vi "set_sweep_period.vi"(8 "error in (no error)":errorcluster, 10 "sweep period":dbl[unit], 11 "DL090130ExperimentController.lvclass in":refnum<class "ExperimentControllerDL090130Interval.lvclass">) -> (0 "error out":errorcluster, 3 "DL090130ExperimentController.lvclass out":refnum<class "ExperimentControllerDL090130Interval.lvclass">)   [LabVIEW 2010, in "ExperimentControllerDL090130Interval.lvclass"]
uses:
  ExperimentControllerDL090130Interval.lvclass
  ExperimentControllerDL090130Interval.lvclass/ExperimentControllerDL090130Interval.ctl
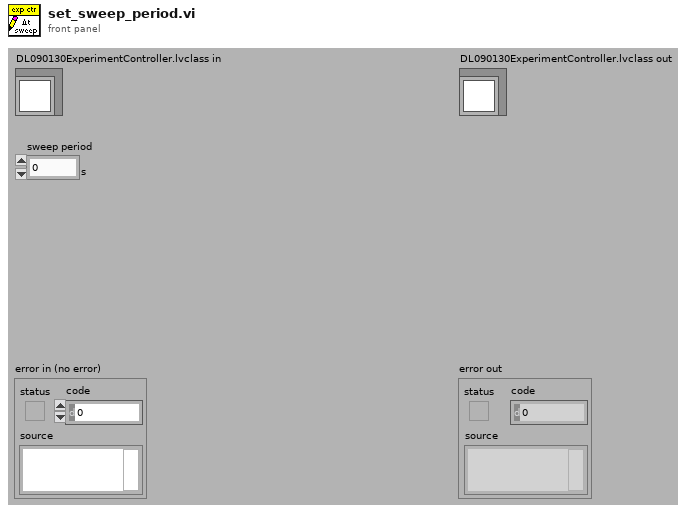
[diagram p1: front panel]
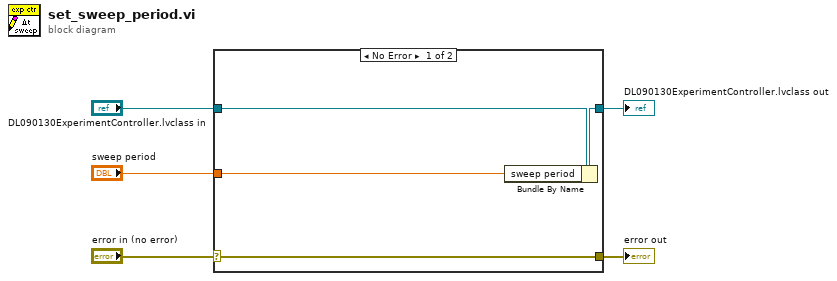
[diagram p0: block diagram]
diagram:
  n1 = case shown="No Error" "error in (no error)" {
    selector: "error in (no error)" -> [w9 w10]
    tunnel: [w9 w10] -> w4
    tunnel: [w7 w11] -> w2
    tunnel: "DL090130ExperimentController.lvclass in" -> [w8 w11]
    tunnel: "sweep period" -> [w6 _]
    frame No Error {
      n2 = Bundle By Name(cluster=w8, "sweep period"=w6) -> (w7:refnum<class "ExperimentControllerDL090130Interval.lvclass">)
    }
    frame Error {
    }
  }
  "error out" <- w4
  "DL090130ExperimentController.lvclass out" <- w2
